vi "test-slew-rate-limiter-demo.vi"() -> ()   [LabVIEW 2019]
uses:
  <vilib>/Rock Robotics/WPI/ThirdParty/JAS_Junk/TrajLib/Trajectory_Library.lvlib
panel:
  in  "Rate Limit":dbl=9999.0
  out "Waveform Chart":cluster{dbl, dbl}(graph)
  in  "Frequency":dbl(slide)=0.2 min=0.1 max=1000.0 step=0.5 scale=0.1..10.0
  in  "Amplitude":dbl(slide)=1.0 scale=0.0..10.0
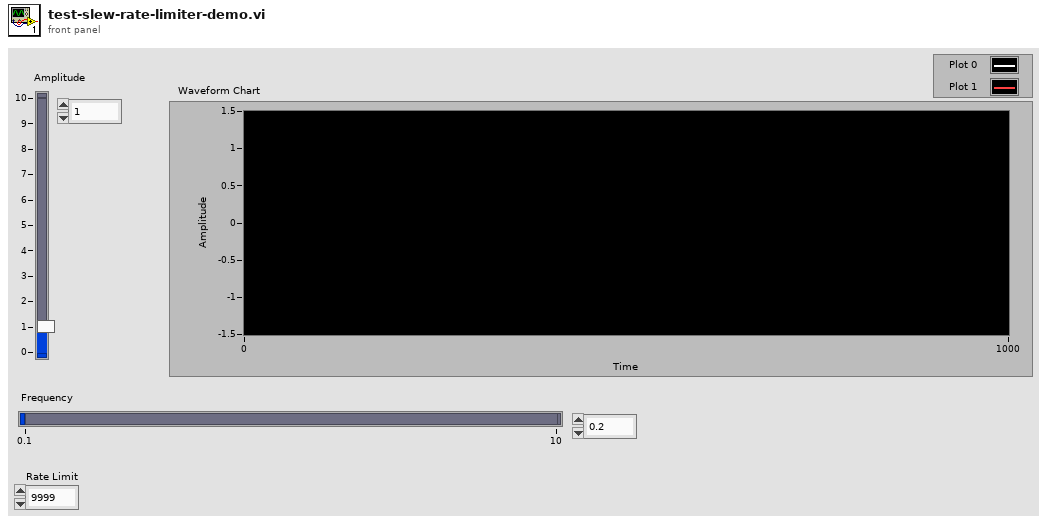
[diagram p1: front panel]
types:
  T1 = typedef "Trajectory_Library.lvlib/SLEW_RATE_LIMITER.ctl" = cluster{"RateLimit":dbl, "PrevValue":dbl, "PrevTime":dbl}
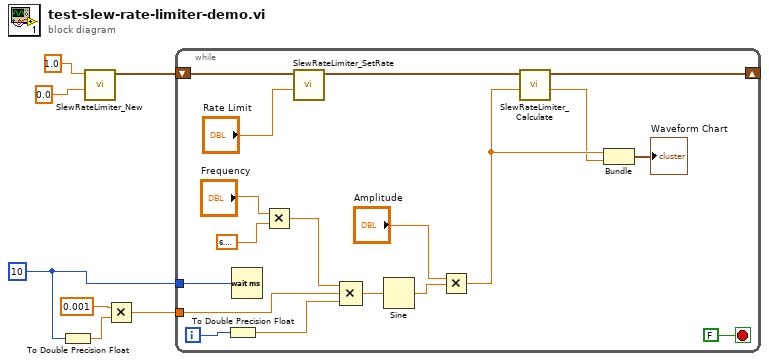
[diagram p0: block diagram]
diagram:
  w4 = u32 10 ("milliseconds to wait")
  n1 = To Double Precision Float(number=w4) -> (double precision float=w5:dbl)
  n2 = call <vilib>:"SlewRateLimiter_New.vi"("InitialValue"=0.0, "RateLimit"=1.0) -> ("out SLEW_RATE_LIMITER"=w1:T1)  [unwired: 9 in]
  n3 = Multiply(x=0.001 ("value"), y=w5) -> (x*y=w3:dbl)
  n4 = while {
    tunnel: w4 -> [w16]
    tunnel: w3 -> [w14]
    shift-right: [w8] -> _
    shift-left: w1 -> [w13]
    i -> [w24]
    stop <- FALSE stop-if-true
    n5 = To Double Precision Float(number=w24) -> (double precision float=w23:dbl)
    n6 = Wait (ms)(milliseconds to wait=w16) -> ()  [unwired: 1 out]
    n7 = Multiply(x="Frequency", y=6.283185307179586) -> (x*y=w15:dbl)
    n8 = call <vilib>:"SlewRateLimiter_SetRate.vi"("Rate"="Rate Limit", "in SLEW_RATE_LIMITER"=w13) -> ("out SLEW_RATE_LIMITER"=w9:T1)  [unwired: 9 in]
    n9 = Compound Arithmetic op=MULTIPLY(w15, w14, w23) -> (w22:dbl)
    n10 = Sine(x=w22) -> (sin(x)=w21:dbl)
    n11 = Multiply(x="Amplitude", y=w21) -> (x*y=w11:dbl)
    n12 = call <vilib>:"SlewRateLimiter_Calculate.vi"("Input"=w11, "in SLEW_RATE_LIMITER"=w9) -> ("Output"=w10:dbl, "out SLEW_RATE_LIMITER"=w8:T1)  [unwired: 8 in]
    n13 = Bundle(w11, "Output"=w10) -> (→"Waveform Chart":cluster{dbl, "Output":dbl})  [unwired: 1 in]
  }
